vi "SRA.vi"(0 "System no.":i32=1 min=1 max=4 step=1, 2 "Axes to set":string[](array[string]), 3 "Gear ratio values":dbl[](array[numeric]) format="%.6f", 4 "No.of digits":i16=4, 5 "error in":errorcluster) -> (19 "error out":errorcluster)   [LabVIEW 2020]
doc: "Sets gear ratio for electronic gearing mode. No. of digits is the number of digits after the decimal point in the gear ratio value(s) that will be sent.\n\nC-843 This command can only be issued to a slave axis. Use MAS to define the master axis.\n\nC-848: This command can only be issued to a slave axis. The master-slave assignments are hardware-dependent.\n\nC-880: This command can only be issued to a slave axis. The master-slave assignments are hardware-dependent."
panel:
  # "Sets gear ratio for electronic gearing mode."
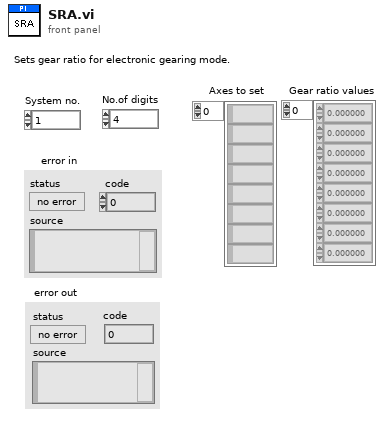
[diagram p1: front panel]
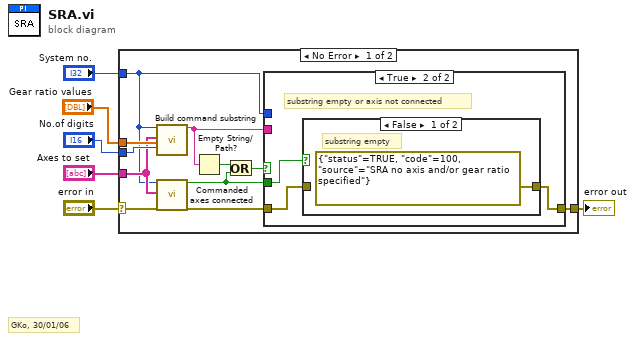
[diagram p0: block diagram]
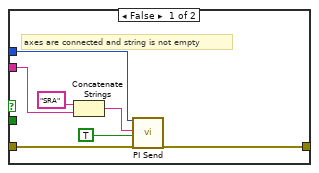
[diagram p2: hidden frame]
diagram:
  # "GKo, 30/01/06"
  n1 = case shown="No Error" "error in" {
    selector: "error in" -> [w7 w30]
    tunnel: [w17 w30] -> w6
    tunnel: "Gear ratio values" -> [w16 _]
    tunnel: "No.of digits" -> [w15 _]
    tunnel: "System no." -> [w11 _]
    tunnel: "Axes to set" -> [w13 _]
    frame No Error {
      n2 = call "Build command substring.vi"("System no."=w11, "Affected axes"=w13, "Parameters"=w16, "No. of digits"=w15) -> ("Command substring"=w9:string)  [unwired: 3 in, 12 out]
      n3 = call "Commanded axes connected.vi"("System no."=w11, "Commanded axes"=w13, "error in"=w7) -> ("Controller error"=w8:bool, "error out"=w14:errorcluster)  [unwired: 1 in, 14 out]
      n4 = Empty String/Path?(string/path=w9) -> (empty?=w10:bool)
      n5 = Or(x=w10, y=w8) -> (x .or. y?=w12:bool)
      n6 = case shown="True" w12 {
        tunnel: w9 -> [w23 _]
        tunnel: [w19 w27] -> w17
        tunnel: w14 -> [w20 w25]
        tunnel: w8 -> [_ w26]
        tunnel: w11 -> [w18 _]
        frame False {
          # "axes are connected and string is not empty"
          n7 = Concatenate Strings("SRA", w23) -> (w21:string)
          n8 = call "PI Send.vi"("System no."=w18, "String to send"=w21, "Attach termination char.?"=TRUE ("Attach Linefeed?"), "error in"=w20) -> ("error out"=w19:errorcluster)  [unwired: 2 in, 13 out]
        }
        frame True {
          # "substring empty or axis not connected"
          n9 = case shown="False" w26 {
            tunnel: [errorcluster {"status"=TRUE, "code"=100, "source"="SRA no axis and/or gear ratio  specified"} ("error out") w29] -> w27
            tunnel: w25 -> [_ w29]
            frame False {
              # "substring empty"
            }
            frame True {
              # "commanded axis\n not connected"
            }
          }
        }
      }
    }
    frame Error {
    }
  }
  "error out" <- w6
